vi "DisplayChunk.vi"(0 "UI Graphs":T1, 2 "Value":T2(ring), 3 "Waveform":waveform(dbl), 4 "MeasureMode":enum32{"RT Monitor", "IV Monitor"}(ring), 6 "Array":waveform(dbl)[](array[waveform])) -> ()   [LabVIEW 2020]
uses:
  C:/Users/bashc/Desktop/ChannelAutomatorR_.06/UIGraphs.ctl
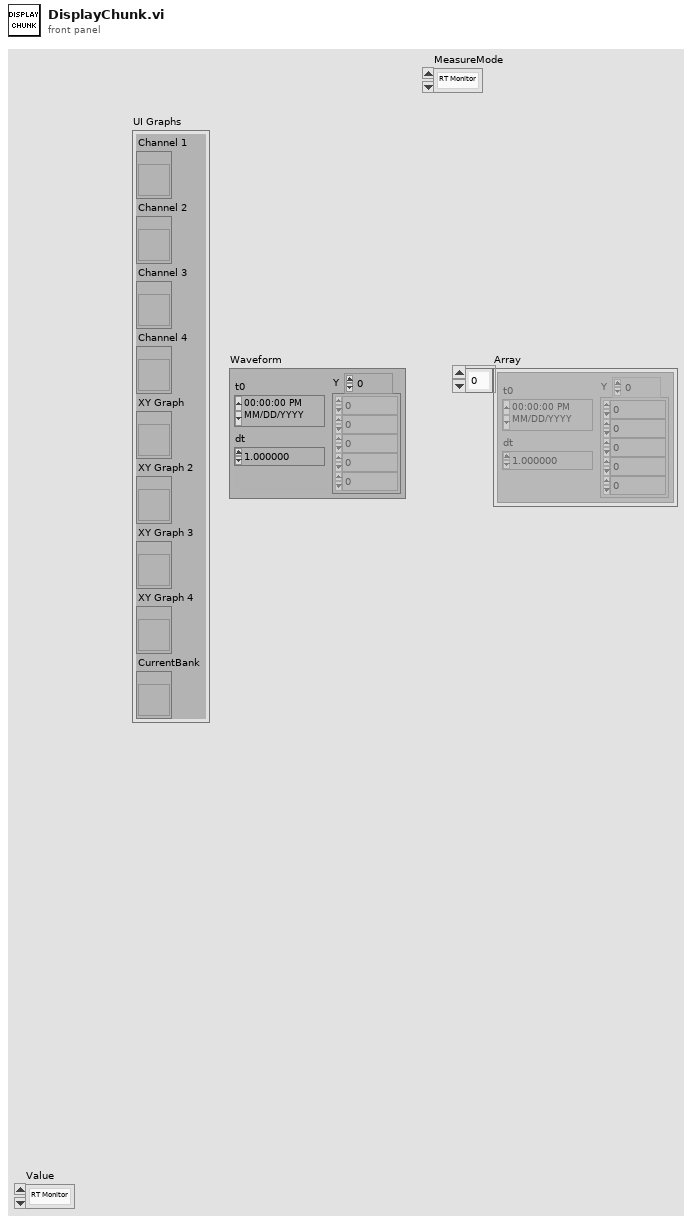
[diagram p1: front panel]
types:
  T1 = typedef "UIGraphs.ctl" = cluster{"Channel 1":refnum<vi>, "Channel 2":refnum<vi>, "Channel 3":refnum<vi>, "Channel 4":refnum<vi>, "XY Graph":refnum<vi>, "XY Graph 2":refnum<vi>, "XY Graph 3":refnum<vi>, "XY Graph 4":refnum<vi>, "CurrentBank":refnum<vi>}
  T2 = enum32{"RT Monitor", "IV Monitor", "View All", "Experiment", "Settings"}
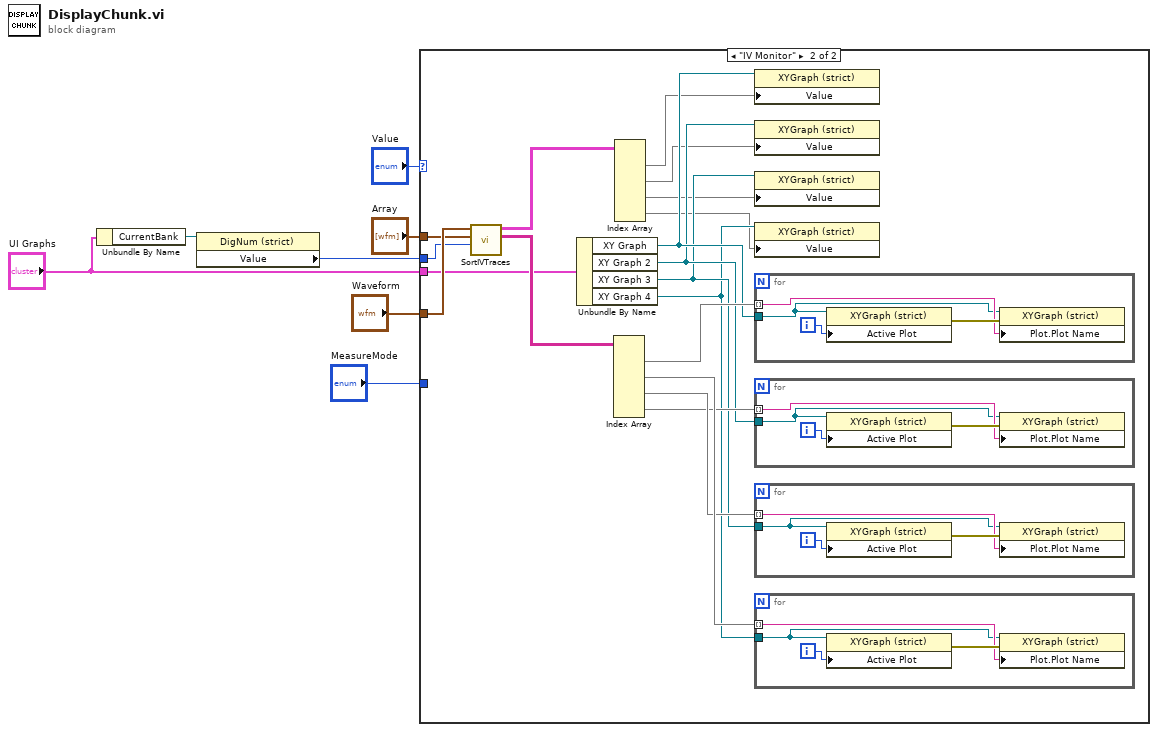
[diagram p0: block diagram]
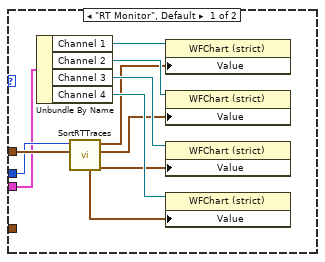
[diagram p2: hidden frame]
diagram:
  n1 = Unbundle By Name("UI Graphs") -> ("CurrentBank"=w3:refnum<vi>)
  n2 = property class="DigNum (strict)"(reference=w3) -> ("Value"=w2:i32)  [unwired: 1 in, 2 out]
  n3 = case shown="\"IV Monitor\"" "Value" {
    tunnel: "Array" -> [w18 w35]
    tunnel: "Waveform" -> [_ w36]
    tunnel: "MeasureMode" -> [_ _]
    tunnel: w2 -> [w17 w28]
    tunnel: "UI Graphs" -> [w16 w27]
    frame "RT Monitor", Default {
      n4 = Unbundle By Name(w16) -> ("Channel 1"=w15:refnum<vi>, "Channel 2"=w14:refnum<vi>, "Channel 3"=w13:refnum<vi>, "Channel 4"=w12:refnum<vi>)
      n5 = call "SortRTTraces.vi"("Array in"=w18, "CurrentBank"=w17) -> ("Array 7"=w9:waveform(dbl)[], "Array 5"=w10:waveform(dbl)[], "Array 6"=w11:waveform(dbl)[], "Array 4"=w8:waveform(dbl)[])  [unwired: 6 in]
      n6 = property class="WFChart (strict)"(reference=w15, "Value"=w11) -> ()  [unwired: 1 in, 2 out]
      n7 = property class="WFChart (strict)"(reference=w14, "Value"=w10) -> ()  [unwired: 1 in, 2 out]
      n8 = property class="WFChart (strict)"(reference=w13, "Value"=w9) -> ()  [unwired: 1 in, 2 out]
      n9 = property class="WFChart (strict)"(reference=w12, "Value"=w8) -> ()  [unwired: 1 in, 2 out]
    }
    frame "IV Monitor" {
      n10 = call "SortIVTraces.vi"("CurrentBank"=w28, "Array in"=w35, "Waveform"=w36) -> ("channelNames"=w33:string[][], "Plots"=w34:cluster{"Y":dbl[], "Y":dbl[]}[][])  [unwired: 7 in]
      n11 = Unbundle By Name(w27) -> ("XY Graph"=w26:refnum<vi>, "XY Graph 2"=w25:refnum<vi>, "XY Graph 3"=w24:refnum<vi>, "XY Graph 4"=w23:refnum<vi>)
      n12 = Index Array(array=w33) -> (element #1=w32:string[], element #2=w31:string[], element #3=w30:string[], element #4=w29:string[])  [unwired: 8 in]
      n13 = Index Array(array=w34) -> (element #1=w22:cluster{"Y":dbl[], "Y":dbl[]}[], element #2=w21:cluster{"Y":dbl[], "Y":dbl[]}[], element #3=w20:cluster{"Y":dbl[], "Y":dbl[]}[], element #4=w19:cluster{"Y":dbl[], "Y":dbl[]}[])  [unwired: 8 in]
      n14 = property class="XYGraph (strict)"(reference=w26, "Value"=w22) -> ()  [unwired: 1 in, 2 out]
      n15 = property class="XYGraph (strict)"(reference=w25, "Value"=w21) -> ()  [unwired: 1 in, 2 out]
      n16 = property class="XYGraph (strict)"(reference=w24, "Value"=w20) -> ()  [unwired: 1 in, 2 out]
      n17 = property class="XYGraph (strict)"(reference=w23, "Value"=w19) -> ()  [unwired: 1 in, 2 out]
      n18 = for {
        tunnel: w32 -> [w51] mode=indexing
        tunnel: w26 -> [w49]
        i -> [w50]
        n19 = property on="Property Node" class="XYGraph (strict)"(reference=w49, "Active Plot"=w50) -> (error out=w52:errorcluster)  [unwired: 1 in, 1 out]
        n20 = property on="Property Node" class="XYGraph (strict)"(reference=w49, error in=w52, "Plot.Plot Name"=w51) -> ()  [unwired: 2 out]
      }
      n21 = for {
        tunnel: w29 -> [w39] mode=indexing
        tunnel: w25 -> [w37]
        i -> [w38]
        n22 = property on="Property Node" class="XYGraph (strict)"(reference=w37, "Active Plot"=w38) -> (error out=w40:errorcluster)  [unwired: 1 in, 1 out]
        n23 = property on="Property Node" class="XYGraph (strict)"(reference=w37, error in=w40, "Plot.Plot Name"=w39) -> ()  [unwired: 2 out]
      }
      n24 = for {
        tunnel: w30 -> [w42] mode=indexing
        tunnel: w24 -> [w41]
        i -> [w43]
        n25 = property on="Property Node" class="XYGraph (strict)"(reference=w41, "Active Plot"=w43) -> (error out=w44:errorcluster)  [unwired: 1 in, 1 out]
        n26 = property on="Property Node" class="XYGraph (strict)"(reference=w41, error in=w44, "Plot.Plot Name"=w42) -> ()  [unwired: 2 out]
      }
      n27 = for {
        tunnel: w31 -> [w46] mode=indexing
        tunnel: w23 -> [w45]
        i -> [w47]
        n28 = property on="Property Node" class="XYGraph (strict)"(reference=w45, "Active Plot"=w47) -> (error out=w48:errorcluster)  [unwired: 1 in, 1 out]
        n29 = property on="Property Node" class="XYGraph (strict)"(reference=w45, error in=w48, "Plot.Plot Name"=w46) -> ()  [unwired: 2 out]
      }
    }
  }
